vi "start.vi"(8 "error in (no error)":errorcluster, 10 "start":bool, 11 "AtomChipHWC in":refnum<class "AtomChipHWC.lvclass">) -> (0 "error out":errorcluster, 2 "started":bool, 3 "AtomChipHWC out":refnum<class "AtomChipHWC.lvclass">)   [LabVIEW 2009, in "Hardware.lvlib" / "HWControllers.lvlib" / "AtomChipHWC.lvclass"]
doc: "Start running an experiment. I.e. Start all hardware."
uses:
  AtomChipHWC.lvclass
  AtomChipHWC.lvclass/AtomChipHWC.ctl
  HardwareConfiguration/HWConfiguration.lvclass
  Channels/Digital/DigitalOutput.lvclass
  Channels/VoltOutput/AnalogOutput.lvclass
  Channels/DDSOutput/Generic/DDSOutput.lvclass
  Tools/Filing/FileNeologist/FileNeologist.lvclass
  HWController.lvclass
  Tools/Filing.lvlib
panel:
  out "time to start":dbl
  # "not used here"
  # "not used here"
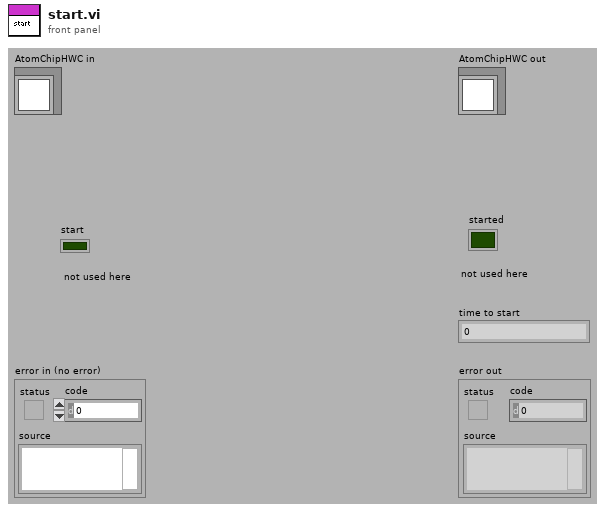
[diagram p1: front panel]
types:
  T1 = enum16{"Ready", "Compiling", "Configured", "Running", "Stopping", "Unresolved Error"}
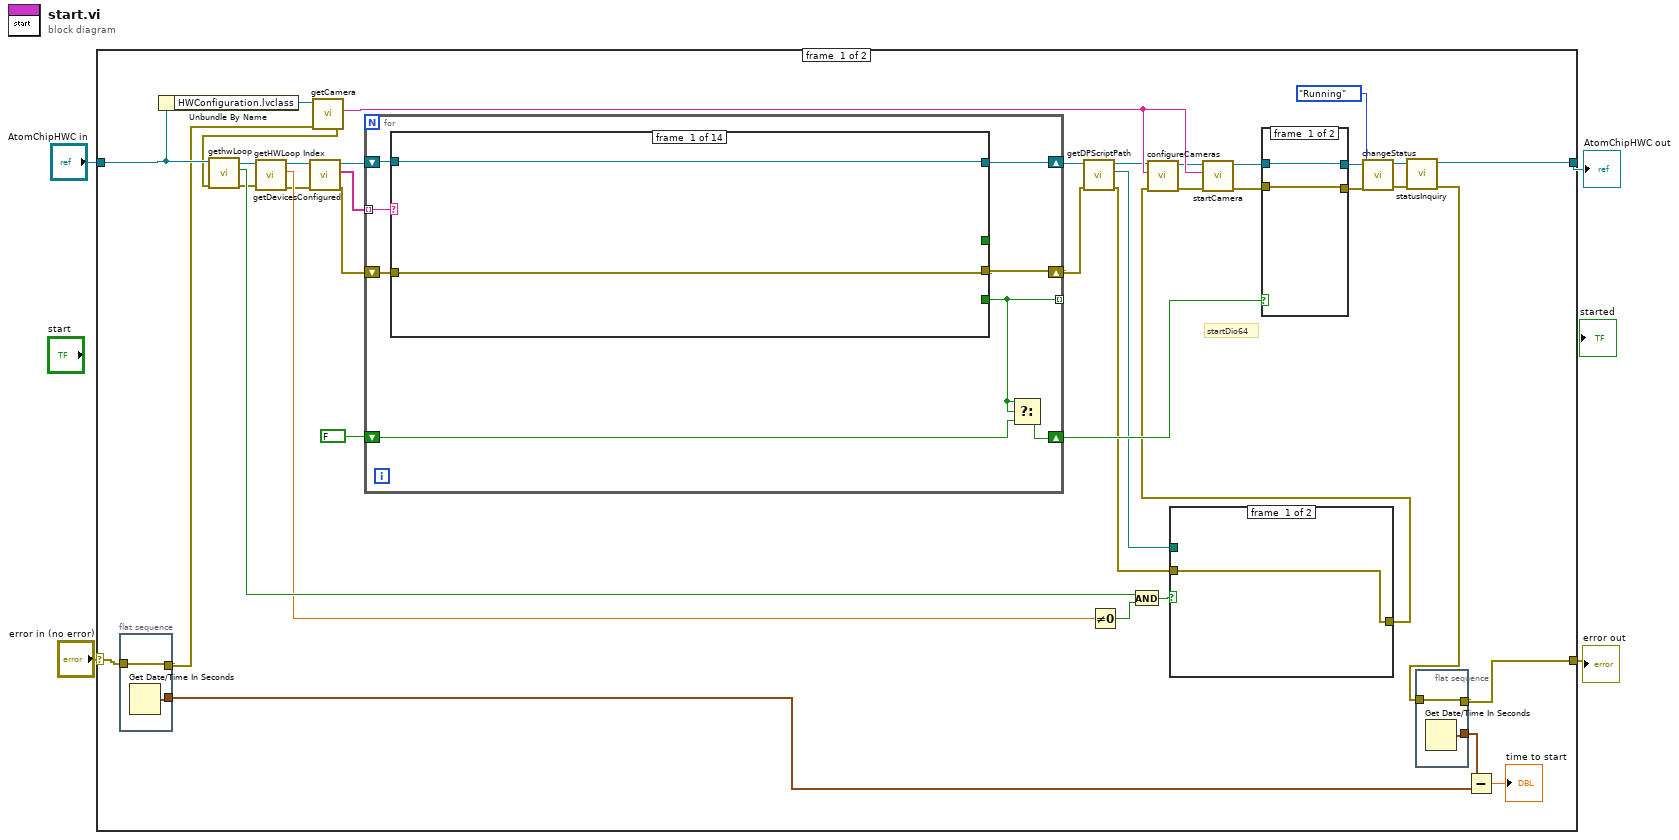
[diagram p0: block diagram]
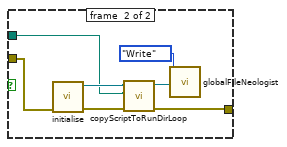
[diagram p2: hidden frame]
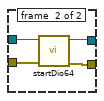
[diagram p3: hidden frame]
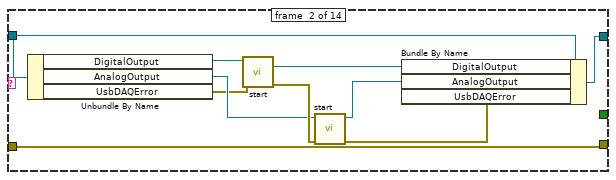
[diagram p4: hidden frame]
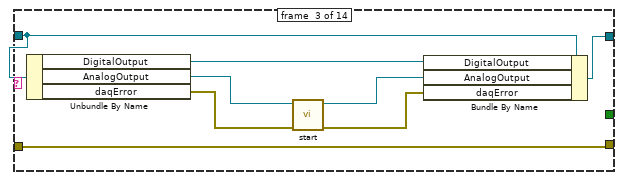
[diagram p5: hidden frame]
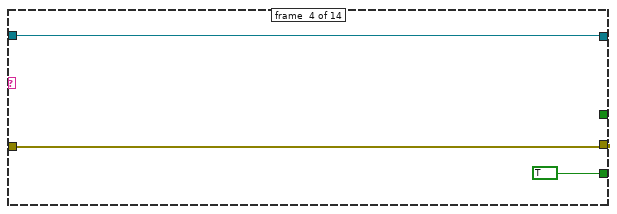
[diagram p6: hidden frame]
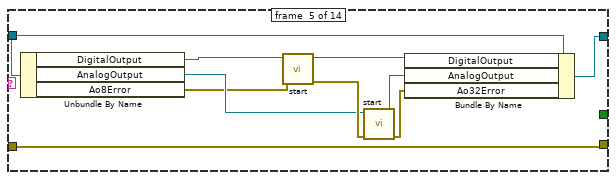
[diagram p7: hidden frame]
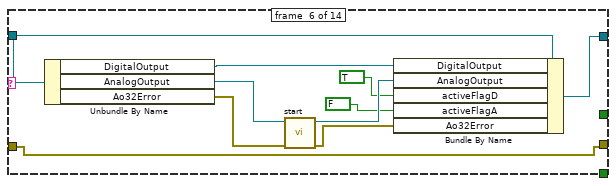
[diagram p8: hidden frame]
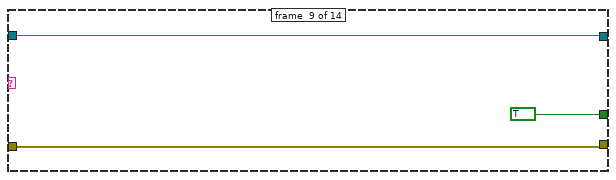
[diagram p11: hidden frame]
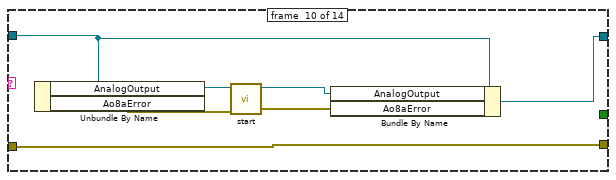
[diagram p12: hidden frame]
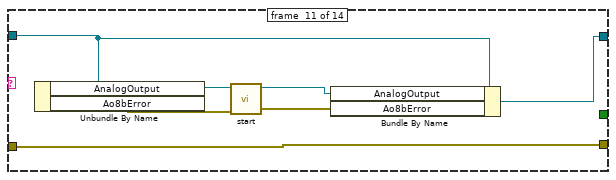
[diagram p13: hidden frame]
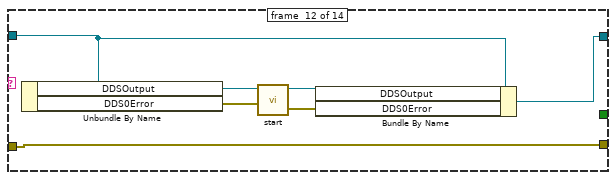
[diagram p14: hidden frame]
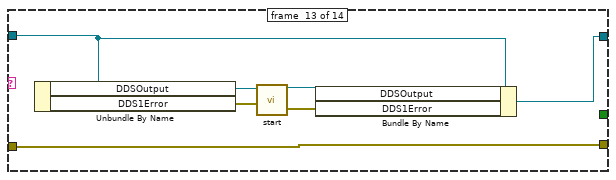
[diagram p15: hidden frame]
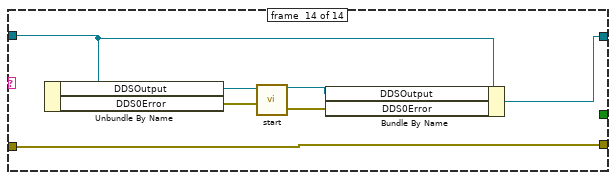
[diagram p16: hidden frame]
diagram:
  n1 = case shown="No Error" "error in (no error)" {
    selector: "error in (no error)" -> [w11 w156]
    tunnel: [w8 w156] -> w3
    tunnel: [w44 w157] -> w1
    tunnel: "AtomChipHWC in" -> [w43 w157]
    frame #0 {
      # "startDio64"
      n2 = flat-sequence {
        tunnel: [w48] -> w10
        tunnel: w11 -> [w48]
        tunnel: [w47] -> w6
        frame #0 {
          n3 = Get Date/Time In Seconds() -> (seconds since 1Jan1904=w47:timestamp)
        }
      }
      n4 = Unbundle By Name(w43) -> ("HWConfiguration.lvclass"=w34:refnum<class "HWConfiguration.lvclass">)
      n5 = call-dynamic "getCamera.vi"("error in (no error)"=w10, "HWConfiguration.lvclass in"=w34) -> ("error out"=w33:errorcluster, "camera"=w24:string)  [unwired: 7 in, 1 out]
      n6 = call "gethwLoop.vi"("error in (no error)"=w33, "HWController in"=w43) -> ("error out"=w30:errorcluster, "hwLoop?"=w32:bool, "HWController out"=w31:refnum<class "AtomChipHWC.lvclass">)  [unwired: 7 in]
      n7 = call "getHWLoop Index.vi"("error in (no error)"=w30, "HWController in"=w31) -> ("error out"=w25:errorcluster, "HWLoop Index"=w29:dbl, "HWController out"=w26:refnum<class "AtomChipHWC.lvclass">)  [unwired: 7 in]
      n8 = call "getDevicesConfigured.vi"("error in (no error)"=w25, "HWController.lvclass in"=w26) -> ("error out"=w37:errorcluster, "devicesConfigured"=w38:string[], "HWController.lvclass out"=w39:refnum<class "AtomChipHWC.lvclass">)  [unwired: 7 in]
      n9 = for {
        tunnel: w38 -> [w69] mode=indexing
        shift-right: [w67] -> w23
        shift-left: w39 -> [w70]
        shift-right: [w66] -> w21
        shift-left: w37 -> [w68]
        tunnel: [w65] -> _ mode=indexing
        shift-right: [w63] -> w42
        shift-left: FALSE -> [w64]
        n10 = case shown="\"CQTDDS0\"" w69 {
          tunnel: [w72 w81 w90 w93 w101 w113 w115 w117 w120 w126 w133 w141 w148 w155] -> w67
          tunnel: [w71 w73 w83 w92 w94 w104 w114 w116 w119 w121 w128 w135 w142 w149] -> w66
          tunnel: w70 -> [w72 w82 w89 w93 w102 w112 w115 w117 w120 w125 w132 w140 w147 w154]
          tunnel: w68 -> [w71 w73 w83 w92 w94 w104 w114 w116 w119 w121 w128 w135 w142 w149]
          tunnel: [_ _ _ TRUE _ _ _ _ _ _ _ _ _ _] -> w65
          tunnel: [_ _ _ _ _ _ _ _ TRUE _ _ _ _ _] -> _
          frame #0 {
          }
          frame #1 {
            n11 = Unbundle By Name(w82) -> ("DigitalOutput"=w79:refnum<class "DigitalOutput.lvclass">, "AnalogOutput"=w78:refnum<class "AnalogOutput.lvclass">, "UsbDAQError"=w74:errorcluster)
            n12 = call-dynamic "start.vi"("error in (no error)"=w74, "DigitalOutput in"=w79) -> ("error out"=w80:errorcluster, "DigitalOutput out"=w77:refnum<class "DigitalOutput.lvclass">)  [unwired: 8 in]
            n13 = call-dynamic "start.vi"("error in (no error)"=w80, "AnalogOutput in"=w78) -> ("error out"=w75:errorcluster, "AnalogOutput out"=w76:refnum<class "AnalogOutput.lvclass">)  [unwired: 8 in]
            n14 = Bundle By Name(cluster=w82, "DigitalOutput"=w77, "AnalogOutput"=w76, "UsbDAQError"=w75) -> (w81:refnum<class "AtomChipHWC.lvclass">)
          }
          frame #2 {
            n15 = Unbundle By Name(w89) -> ("DigitalOutput"=w86:refnum<class "DigitalOutput.lvclass">, "AnalogOutput"=w88:refnum<class "AnalogOutput.lvclass">, "daqError"=w85:errorcluster)
            n16 = call-dynamic "start.vi"("error in (no error)"=w85, "AnalogOutput in"=w88) -> ("error out"=w84:errorcluster, "AnalogOutput out"=w87:refnum<class "AnalogOutput.lvclass">)  [unwired: 8 in]
            n17 = Bundle By Name(cluster=w89, "DigitalOutput"=w86, "AnalogOutput"=w87, "daqError"=w84) -> (w90:refnum<class "AtomChipHWC.lvclass">)
          }
          frame #3 {
          }
          frame #4 {
            n18 = Unbundle By Name(w102) -> ("DigitalOutput"=w100:refnum<class "DigitalOutput.lvclass">, "AnalogOutput"=w97:refnum<class "AnalogOutput.lvclass">, "Ao8Error"=w95:errorcluster)
            n19 = call-dynamic "start.vi"("error in (no error)"=w95, "DigitalOutput in"=w100) -> ("error out"=w103:errorcluster, "DigitalOutput out"=w99:refnum<class "DigitalOutput.lvclass">)  [unwired: 8 in]
            n20 = call-dynamic "start.vi"("error in (no error)"=w103, "AnalogOutput in"=w97) -> ("error out"=w96:errorcluster, "AnalogOutput out"=w98:refnum<class "AnalogOutput.lvclass">)  [unwired: 8 in]
            n21 = Bundle By Name(cluster=w102, "DigitalOutput"=w99, "AnalogOutput"=w98, "Ao32Error"=w96) -> (w101:refnum<class "AtomChipHWC.lvclass">)
          }
          frame #5 {
            n22 = Unbundle By Name(w112) -> ("DigitalOutput"=w109:refnum<class "DigitalOutput.lvclass">, "AnalogOutput"=w111:refnum<class "AnalogOutput.lvclass">, "Ao32Error"=w105:errorcluster)
            n23 = call-dynamic "start.vi"("error in (no error)"=w105, "AnalogOutput in"=w111) -> ("error out"=w106:errorcluster, "AnalogOutput out"=w110:refnum<class "AnalogOutput.lvclass">)  [unwired: 8 in]
            n24 = Bundle By Name(cluster=w112, "DigitalOutput"=w109, "AnalogOutput"=w110, "activeFlagD"=TRUE, "activeFlagA"=FALSE, "Ao32Error"=w106) -> (w113:refnum<class "AtomChipHWC.lvclass">)
          }
          frame #6 {
          }
          frame #7 {
          }
          frame #8 {
          }
          frame #9 {
            n25 = Unbundle By Name(w125) -> ("AnalogOutput"=w127:refnum<class "AnalogOutput.lvclass">, "Ao8aError"=w123:errorcluster)
            n26 = call-dynamic "start.vi"("error in (no error)"=w123, "AnalogOutput in"=w127) -> ("error out"=w122:errorcluster, "AnalogOutput out"=w124:refnum<class "AnalogOutput.lvclass">)  [unwired: 8 in]
            n27 = Bundle By Name(cluster=w125, "AnalogOutput"=w124, "Ao8aError"=w122) -> (w126:refnum<class "AtomChipHWC.lvclass">)
          }
          frame #10 {
            n28 = Unbundle By Name(w132) -> ("AnalogOutput"=w134:refnum<class "AnalogOutput.lvclass">, "Ao8bError"=w130:errorcluster)
            n29 = call-dynamic "start.vi"("error in (no error)"=w130, "AnalogOutput in"=w134) -> ("error out"=w129:errorcluster, "AnalogOutput out"=w131:refnum<class "AnalogOutput.lvclass">)  [unwired: 8 in]
            n30 = Bundle By Name(cluster=w132, "AnalogOutput"=w131, "Ao8bError"=w129) -> (w133:refnum<class "AtomChipHWC.lvclass">)
          }
          frame #11 {
            n31 = Unbundle By Name(w140) -> ("DDSOutput"=w139:refnum<class "DDSOutput.lvclass">, "DDS0Error"=w137:errorcluster)
            n32 = call-dynamic "start.vi"("error in (no error)"=w137, "DDSOutput in"=w139) -> ("error out"=w136:errorcluster, "DDSOutput out"=w138:refnum<class "DDSOutput.lvclass">)  [unwired: 8 in]
            n33 = Bundle By Name(cluster=w140, "DDSOutput"=w138, "DDS0Error"=w136) -> (w141:refnum<class "AtomChipHWC.lvclass">)
          }
          frame #12 {
            n34 = Unbundle By Name(w147) -> ("DDSOutput"=w146:refnum<class "DDSOutput.lvclass">, "DDS1Error"=w144:errorcluster)
            n35 = call-dynamic "start.vi"("error in (no error)"=w144, "DDSOutput in"=w146) -> ("error out"=w143:errorcluster, "DDSOutput out"=w145:refnum<class "DDSOutput.lvclass">)  [unwired: 8 in]
            n36 = Bundle By Name(cluster=w147, "DDSOutput"=w145, "DDS1Error"=w143) -> (w148:refnum<class "AtomChipHWC.lvclass">)
          }
          frame #13 {
            n37 = Unbundle By Name(w154) -> ("DDSOutput"=w153:refnum<class "DDSOutput.lvclass">, "DDS0Error"=w151:errorcluster)
            n38 = call-dynamic "start.vi"("error in (no error)"=w151, "DDSOutput in"=w153) -> ("error out"=w150:errorcluster, "DDSOutput out"=w152:refnum<class "DDSOutput.lvclass">)  [unwired: 8 in]
            n39 = Bundle By Name(cluster=w154, "DDSOutput"=w152, "DDS0Error"=w150) -> (w155:refnum<class "AtomChipHWC.lvclass">)
          }
        }
        n40 = Select(t=w65, s=w65, f=w64) -> (s? t:f=w63:bool)
      }
      n41 = call "getDPScriptPath.vi"("error in (no error)"=w21, "HWController in"=w23) -> ("error out"=w19:errorcluster, "DPScriptPath"=w20:path, "HWController out"=w22:refnum<class "AtomChipHWC.lvclass">)  [unwired: 7 in]
      n42 = Not Equal To 0?(x=w29) -> (x != 0?=w28:bool)
      n43 = And(x=w32, y=w28) -> (x .and. y?=w27:bool)
      n44 = case shown="True" w27 {
        tunnel: w19 -> [w49 w55]
        tunnel: w20 -> [_ w51]
        tunnel: [w49 w53] -> w18
        frame #0 {
        }
        frame #1 {
          n45 = call "initialise.vi"("error in (no error)"=w55) -> ("error out"=w54:errorcluster, "FileNeologist out"=w52:refnum<class "FileNeologist.lvclass">)  [unwired: 9 in]
          n46 = call-dynamic "copyScriptToRunDirLoop.vi"("error in (no error)"=w54, "Path in"=w51, "FileNeologist in"=w52) -> ("error out"=w53:errorcluster, "FileNeologist out"=w50:refnum<class "FileNeologist.lvclass">)  [unwired: 6 in, 1 out]
          n47 = call "globalFileNeologist.vi"("FileNeologist in"=w50, "Action"=enum16{"Write", "Read"}."Write") -> ()  [unwired: 9 in, 1 out]
        }
      }
      n48 = call "configureCameras.vi"("error in (no error)"=w18, "deviceName"=w24, "AtomChipHWC in"=w22) -> ("error out"=w16:errorcluster, "AtomChipHWC out"=w17:refnum<class "AtomChipHWC.lvclass">)  [unwired: 7 in]
      n49 = call "startCamera.vi"("error in (no error)"=w16, "camera"=w24, "AtomChipHWC in"=w17) -> ("error out"=w14:errorcluster, "AtomChipHWC out"=w15:refnum<class "AtomChipHWC.lvclass">)  [unwired: 7 in]
      n50 = case shown="True" w42 {
        tunnel: w15 -> [w58 w62]
        tunnel: [w58 w61] -> w13
        tunnel: w14 -> [w57 w60]
        tunnel: [w57 w59] -> w12
        frame #0 {
        }
        frame #1 {
          n51 = call "startDio64.vi"("error in (no error)"=w60, "AtomChipHWC in"=w62) -> ("error out"=w59:errorcluster, "AtomChipHWC out"=w61:refnum<class "AtomChipHWC.lvclass">)  [unwired: 8 in]
        }
      }
      n52 = call "changeStatus.vi"("error in (no error)"=w12, "status"=T1."Running", "HWController in"=w13) -> ("error out"=w40:errorcluster, "HWController out"=w41:refnum<class "AtomChipHWC.lvclass">)  [unwired: 7 in]
      n53 = call-dynamic "statusInquiry.vi"("error in (no error)"=w40, "HWController in"=w41) -> ("error out"=w9:errorcluster, "HWController out"=w44:refnum<class "AtomChipHWC.lvclass">)  [unwired: 8 in]
      n54 = flat-sequence {
        tunnel: [w46] -> w8
        tunnel: w9 -> [w46]
        tunnel: [w45] -> w7
        frame #0 {
          n55 = Get Date/Time In Seconds() -> (seconds since 1Jan1904=w45:timestamp)
        }
      }
      n56 = Subtract(x=w7, y=w6) -> (x-y=→"time to start":dbl)
    }
    frame #1 {
    }
  }
  "error out" <- w3
  "AtomChipHWC out" <- w1
